vi "main.vi"() -> ()   [LabVIEW 2020]
uses:
  TypeDef/display.ctl
  TypeDef/tiles.ctl
  TypeDef/tiles-key.ctl
panel:
  in  "Editor Button":bool
  in  "Play Button":bool
  in  "Settings Button":bool
  in  "Help Button":bool
  out "Display":T1
  in  "stop":bool
  # "Snake"
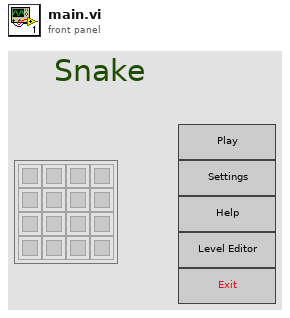
[diagram p1: front panel]
types:
  T1 = typedef "display.ctl" = T2[][]
  T2 = typedef "tiles.ctl" = u16
  T3 = typedef "tiles-key.ctl" = enum16{"ground", "wall", "head (right)", "head (up)", "head (left)", "head (down)", "L-turn (right-up)", "L-turn (up-left)", "L-turn (left-down)", "L-turn (down-right)", "body (right)", "body (up)", "body (left)", "body (down)", "R-turn (right-down)", "R-turn (up-right)", "R-turn (left-up)", "R-turn (down-left)", "tail (right)", "tail (up)", "tail (left)", "tail (down)", "dead head (right)", "dead head (up)", "dead head (left)", "dead head (down)", "dead L-turn (right-up)", "dead L-turn (up-left)", "dead L-turn (left-down)", "dead L-turn (down-right)", "dead body (right)", "dead body (up)", "dead body (left)", "dead body (down)", "dead R-turn (right-down)", "dead R-turn (up-right)", "dead R-turn (left-up)", "dead R-turn (down-left)", "dead tail (right)", "dead tail (up)", "dead tail (left)", "dead tail (down)", "target red", "target blue", "target yellow", "target green"}
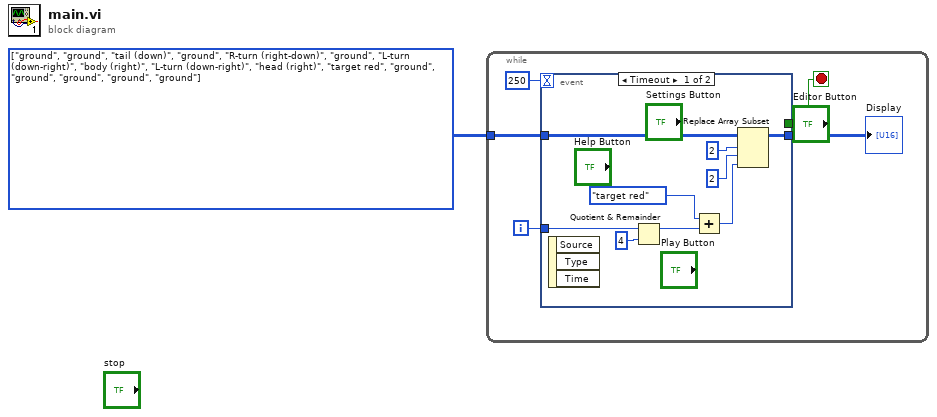
[diagram p0: block diagram]
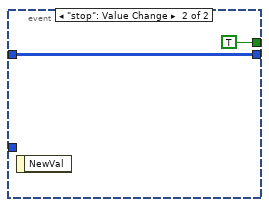
[diagram p2: hidden frame]
diagram:
  w1 = T3[][] [[enum."ground", enum."ground", enum."tail (down)", enum."ground"], [enum."R-turn (right-down)", enum."ground", enum."L-turn (down-right)", enum."body (right)"], [enum."L-turn (down-right)", enum."head (right)", enum."target red", enum."ground"], [enum."ground", enum."ground", enum."ground", enum."ground"]] items=["ground", "wall", "head (right)", "head (up)", "head (left)", "head (down)", "L-turn (right-up)", "L-turn (up-left)", "L-turn (left-down)", "L-turn (down-right)", "body (right)", "body (up)", "body (left)", "body (down)", "R-turn (right-down)", "R-turn (up-right)", "R-turn (left-up)", "R-turn (down-left)", "tail (right)", "tail (up)", "tail (left)", "tail (down)", "dead head (right)", "dead head (up)", "dead head (left)", "dead head (down)", "dead L-turn (right-up)", "dead L-turn (up-left)", "dead L-turn (left-down)", "dead L-turn (down-right)", "dead body (right)", "dead body (up)", "dead body (left)", "dead body (down)", "dead R-turn (right-down)", "dead R-turn (up-right)", "dead R-turn (left-up)", "dead R-turn (down-left)", "dead tail (right)", "dead tail (up)", "dead tail (left)", "dead tail (down)", "target red", "target blue", "target yellow", "target green"] ("Array")
  n1 = while {
    tunnel: w1 -> [w5]
    i -> [w3]
    stop <- w6 stop-if-true
    n2 = event shown="[0] Timeout" {
      selector: _ -> [_ _]
      dyn-events: _ -> [_ _]
      timeout: 250 -> [_ _]
      tunnel: [_ TRUE] -> w6
      tunnel: [w10 w16] -> w2
      tunnel: w5 -> [w15 w16]
      tunnel: w3 -> [w14 _]
      event Timeout {
        n3 = event-data() -> ()  [unwired: 1 in, 3 out]
        n4 = Quotient & Remainder(x=w14, y=4) -> (x-y*floor(x/y)=w12:i32)  [unwired: 1 out]
        n5 = Add(x=tiles-key."target red" ("Tiles-key"), y=w12) -> (x+y=w9:i32)
        n6 = Replace Array Subset(array=w15, new element=w9, index (row)=2, index (col)=2 ("disabled index (col)")) -> (w10:T3[][])
      }
      event "stop": Value Change {
        n7 = event-data() -> ()  [unwired: 1 in, 1 out]
      }
    }
    "Display" <- w2
  }
